vi "m1m3_getEvent_AirSupplyStatus.vi"(8 "error in (no error)":errorcluster, 11 "logevent_AirSupplyStatus_Ctl":T1) -> (0 "error out":errorcluster, 2 "function return":i32, 3 "logevent_AirSupplyStatus_Ctl out":T1)   [LabVIEW 2016, in "SALLV_m1m3.lvlib"]
doc: "int m1m3_shm_getEvent_AirSupplyStatusLV(m1m3_logevent_AirSupplyStatusLV *logevent_AirSupplyStatus_Ctl );"
uses:
  SALLV_m1m3.lvlib
  DataTypes/logevent_AirSupplyStatus.ctl
  SALLV_m1m3.so
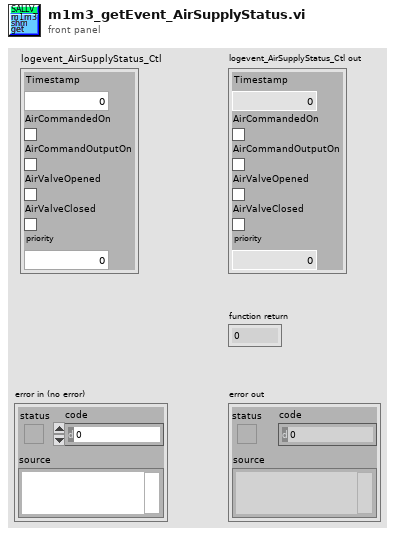
[diagram p1: front panel]
types:
  T1 = typedef "SALLV_m1m3.lvlib/logevent_AirSupplyStatus.ctl" = cluster{"Timestamp":dbl, "AirCommandedOn":bool, "AirCommandOutputOn":bool, "AirValveOpened":bool, "AirValveClosed":bool, "priority":i32}
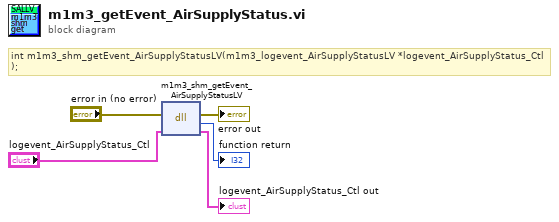
[diagram p0: block diagram]
diagram:
  # "int m1m3_shm_getEvent_AirSupplyStatusLV(m1m3_logevent_AirSupplyStatusLV *logevent_AirSupplyStatus_Ctl );"
  n1 = dll-call lib="opt/CODE/SALLV_m1m3/SALLV_m1m3.*" fn="m1m3_shm_getEvent_AirSupplyStatusLV"(error in="error in (no error)", "logevent_AirSupplyStatus_Ctl"="logevent_AirSupplyStatus_Ctl") -> (error out=→"error out":errorcluster, →"function return":i32, "logevent_AirSupplyStatus_Ctl"=→"logevent_AirSupplyStatus_Ctl out":T1)  [unwired: 2 in, 1 out]
